vi "init_dcam_sCMOS.vi"() -> (0 "error out":errorcluster, 3 "Handle out":u32)   [LabVIEW 2015]
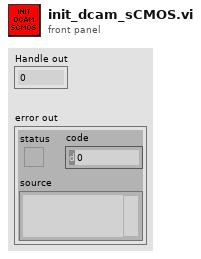
[diagram p1: front panel]
types:
  T1 = cluster{"Mode":u32, "Polarity":u32, "Period":dbl, "Delay":dbl}
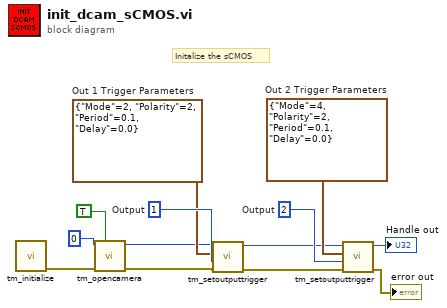
[diagram p0: block diagram]
diagram:
  w7 = T1 {"Mode"=4, "Polarity"=2, "Period"=0.1, "Delay"=0.0}  # Out 2 Trigger Parameters
  w8 = T1 {"Mode"=2, "Polarity"=2, "Period"=0.1, "Delay"=0.0}  # Out 1 Trigger Parameters
  w9 = 2  # Output
  w10 = 1  # Output
  # "Initalize the sCMOS"
  n1 = call <userlib>:"tm_initialize.vi"() -> ("error out"=w13:errorcluster)  [unwired: 8 in, 3 out]
  n2 = call <userlib>:"tm_opencamera.vi"("Force Open"=TRUE, "error in (no error)"=w13, "Camera Index"=0) -> ("error out"=w4:errorcluster, "Handle out"=w3:u32)  [unwired: 6 in, 1 out]
  n3 = call <userlib>:"tm_setoutputtrigger.vi"("error in (no error)"=w4, "Index"=w10, "Parameters"=w8, "Handle in"=w3) -> ("error out"=w6:errorcluster, "Handle out"=w5:u32)  [unwired: 6 in]
  n4 = call <userlib>:"tm_setoutputtrigger.vi"("error in (no error)"=w6, "Index"=w9, "Parameters"=w7, "Handle in"=w5) -> ("error out"=→"error out":errorcluster, "Handle out"=→"Handle out":u32)  [unwired: 6 in]
